vi "initialise.vi"(10 "depth":u32) -> (3 "buffer state":T1)   [LabVIEW 2010, in "OnBoardBuffer.lvlib"]
uses:
  OnBoardBuffer.lvlib
  buffer_state_cluster.ctl
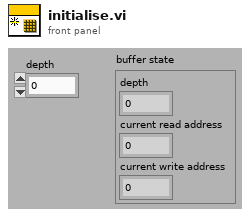
[diagram p1: front panel]
types:
  T1 = typedef "OnBoardBuffer.lvlib/buffer_state_cluster.ctl" = cluster{"depth":u32, "current read address":u32, "current write address":u32}
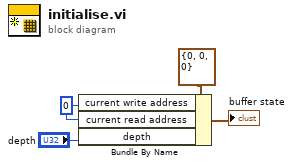
[diagram p0: block diagram]
diagram:
  w3 = u32 0 ("current write address")
  n1 = Bundle By Name(cluster=T1 {"depth"=0, "current read address"=0, "current write address"=0} ("on-board buffer out"), "current write address"=w3, "current read address"=w3, "depth"="depth") -> (→"buffer state":T1)
